vi "CLD 1 Elapsed Time Express Front Panel.vi"() -> ()   [LabVIEW 2018]
doc: "LabVIEW CLD 1 Exercise"
panel:
  out "Elapsed Time (s)":dbl format="%#.0g"
  out "error out":errorcluster
  in  "error in":errorcluster
  out "Time has Elapsed":bool
  in  "Auto Reset":bool=TRUE
  in  "Reset Button":bool
  in  "Stop VI":bool
  in  "Time Target (s)":dbl=2.0
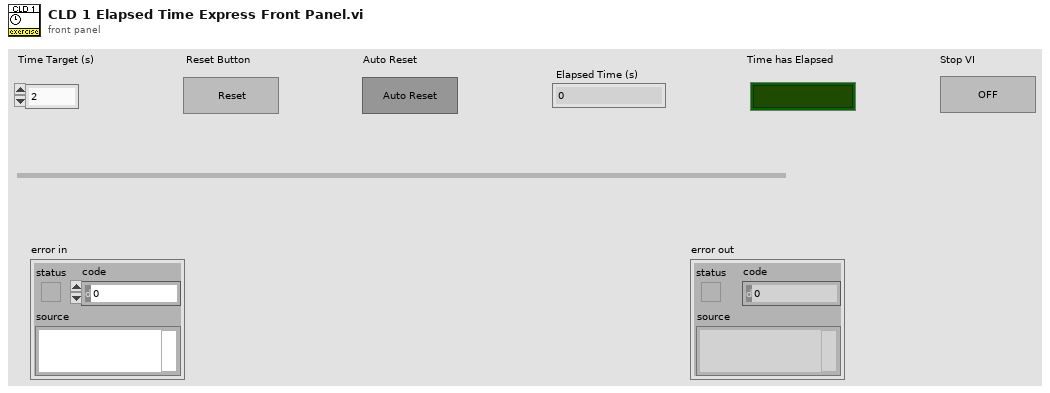
[diagram p1: front panel]
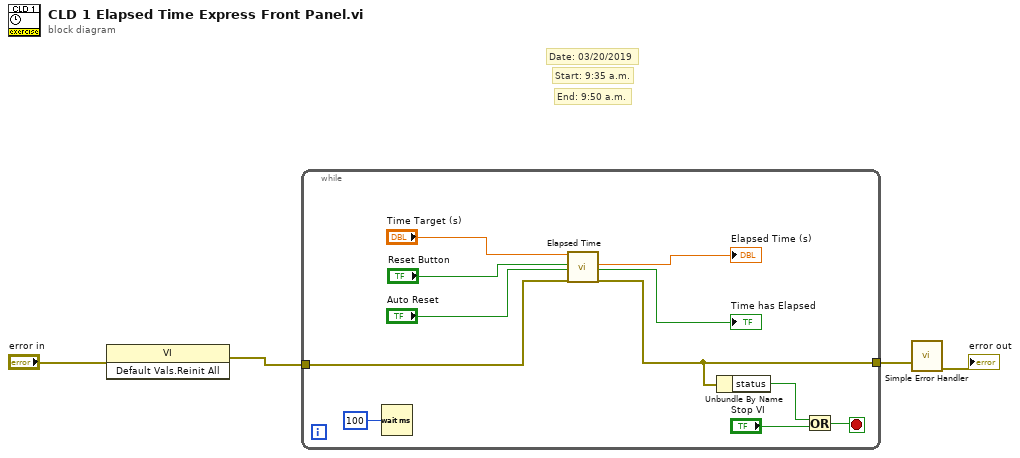
[diagram p0: block diagram]
diagram:
  # "Start: 9:35 a.m."
  # "Date: 03/20/2019"
  # "End: 9:50 a.m."
  n1 = invoke class="VI" method="Default Vals.Reinit All"(error in="error in") -> (error out=w3:errorcluster)  [unwired: 2 in, 2 out]
  n2 = while {
    tunnel: w3 -> [w12]
    tunnel: [w6] -> w2
    stop <- w8 stop-if-true
    n3 = Wait (ms)(milliseconds to wait=u32 100) -> ()  [unwired: 1 out]
    n4 = call "Elapsed Time"("Time Target (s)"="Time Target (s)", "Reset"="Reset Button", "Auto Reset"="Auto Reset", "error in (no error)"=w12) -> ("Elapsed Time (s)"=→"Elapsed Time (s)":dbl, "Time has Elapsed"=→"Time has Elapsed":bool, "error out"=w6:errorcluster)  [unwired: 8 in, 5 out]
    n5 = Unbundle By Name(w6) -> ("status"=w5:bool)
    n6 = Or(x=w5, y="Stop VI") -> (x .or. y?=w8:bool)
  }
  n7 = call <vilib>:"Simple Error Handler.vi"("error in (no error)"=w2) -> ("error out"=→"error out":errorcluster)  [unwired: 4 in, 4 out]
